vi "Resample N Waveforms (single shot, t0 DBL).vi"(0 "waveforms in":waveform(dbl)[](array[waveform]), 1 "open interval? (T)":bool=TRUE, 5 "dt":dbl=1.0 format="%.2p", 7 "t0":dbl=-inf format="%.2p", 9 "interpolation mode":u16(ring)=1 items=["coerce", "linear", "spline", "FIR filter"], 11 "error in (no error)":errorcluster, 12 "FIR filter specifications":T1={"alias rejection (dB)"=120.0, "normalized bandwidth"=0.4536} {"normalized bandwidth" format="%.4f"; "alias rejection (dB)" format="%.2f"}) -> (4 "resampled waveforms out":waveform(dbl)[](array[waveform]), 10 "used t0's":dbl[](array[numeric]) format="%.2p", 14 "t0 adjusted warnings":bool[](array[boolean]), 15 "error out":errorcluster)   [LabVIEW 2020, in "NI_MAPro.lvlib"]
doc: "Resamples input waveforms or data according to the user-defined <B>t0</B> and <B>dt</B> values. You can use this polymorphic VI to resample a single waveform, N waveforms, an array of XY pairs, a pair of X and Y arrays, N arrays of XY pairs, or N pairs of X and Y arrays. The data type you wire to the waveform or data input determines the polymorphic instance to use."
uses:
  NI_MAPro.lvlib
panel:
  # "open"
  # "closed"
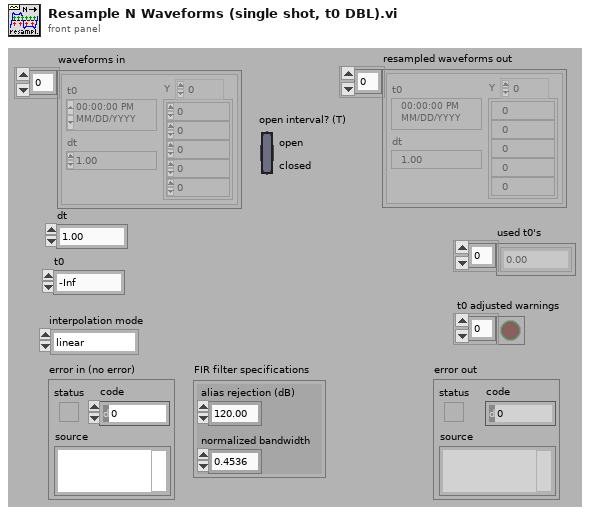
[diagram p1: front panel]
types:
  T1 = cluster{"alias rejection (dB)":dbl, "normalized bandwidth":dbl}
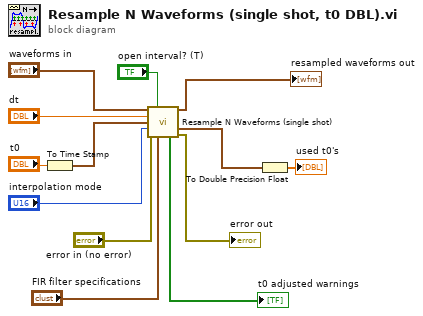
[diagram p0: block diagram]
diagram:
  n1 = To Time Stamp(1:"t0") -> (0:w9:timestamp)
  n2 = call "Resample N Waveforms (single shot).vi"("waveforms in"="waveforms in", "open interval? (F)"="open interval? (T)", "dt"="dt", "t0"=w9, "interpolation mode"="interpolation mode", "error in (no error)"="error in (no error)", "FIR filter specifications"="FIR filter specifications") -> ("resampled waveforms out"=→"resampled waveforms out":waveform(dbl)[], "used t0's"=w2:timestamp[], "t0 adjusted warnings"=→"t0 adjusted warnings":bool[], "error out"=→"error out":errorcluster)  [unwired: 5 in]
  n3 = To Double Precision Float(number=w2) -> (double precision float=→"used t0's":dbl[])
